vi "init_memtest_1channel_justNoise_v02.vi"(6 "memtest":T1={"Samples to Read"=2000, "Rate (Hz)"=20000.0, "Amplitude (mV/pA)"=10.0, "Offset (mV/pA)"=0.0, "Frequency (Hz)"=10.0, "duty cycle (%)"=50.0, "phase"=90.0} {"phase" format="%.2p"; "duty cycle (%)" format="%0.2f"}, 8 "AO error in":errorcluster, 9 "AO physical channels":tag="cDAQ1Mod3/ao14", 10 "AI error in":errorcluster, 11 "AI Physical Channels":tag="cDAQ1Mod1/ai0") -> (0 "AO error out":errorcluster, 1 "AO task out":refnum<k21>, 2 "AI error out":errorcluster, 3 "AI task out":refnum<k21>, 4 "view memtest":waveform(dbl)(graph))   [LabVIEW 2015]
uses:
  <vilib>/DAQmx/configure/timing.llb/DAQmx Timing (Sample Clock).vi
  <vilib>/DAQmx/create/channels.llb/DAQmx Create Channel (AI-Voltage-Basic).vi
  <vilib>/DAQmx/create/channels.llb/DAQmx Create Channel (AO-Voltage-Basic).vi
  <vilib>/DAQmx/configure/trigger.llb/DAQmx Start Trigger (Digital Edge).vi
  <vilib>/DAQmx/write.llb/DAQmx Write (Analog Wfm 1Chan NSamp).vi
  controls/memtest_def.ctl
panel:
  out "command memtest 2":waveform(dbl)(graph)
  out "command memtest":waveform(dbl)(graph)
  in  "which clamp":enum16{"VClamp", "IClamp"}(ring)
  # "init memtest"
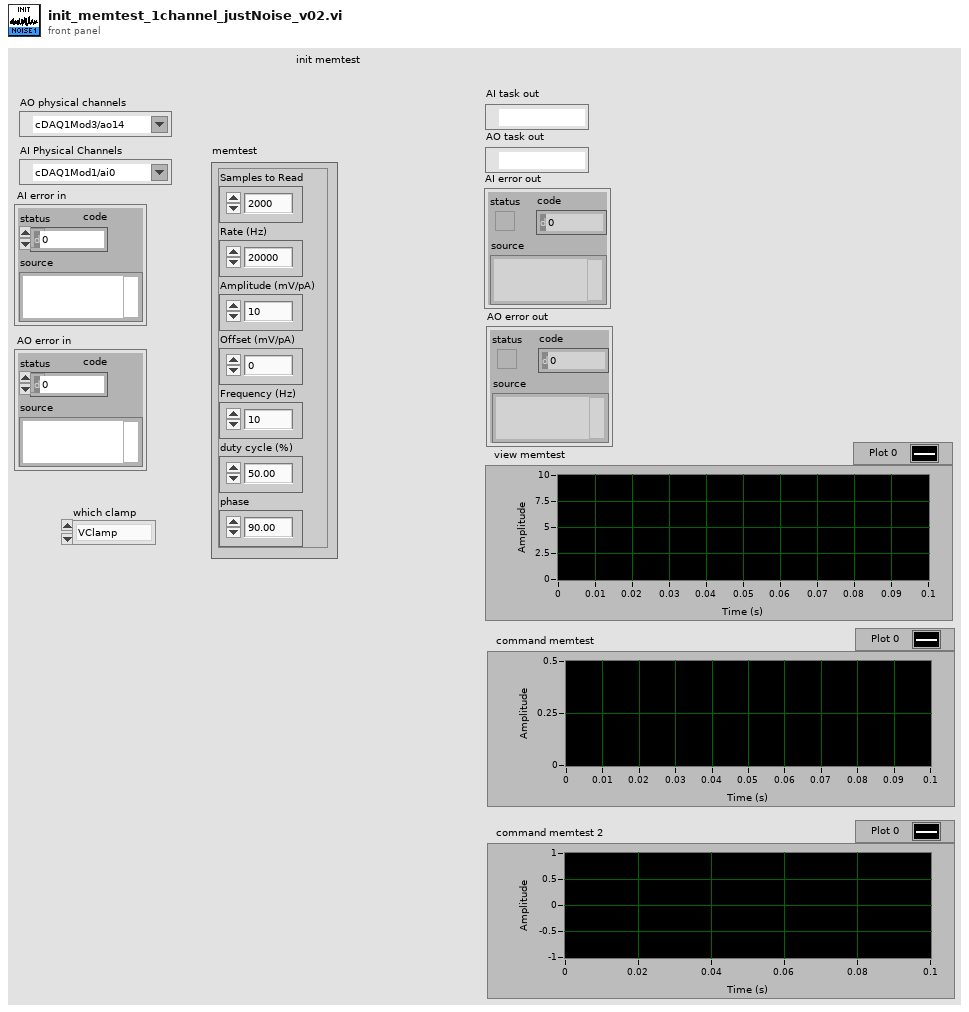
[diagram p1: front panel]
types:
  T1 = typedef "memtest_def.ctl" = cluster{"Samples to Read":i32, "Rate (Hz)":dbl, "Amplitude (mV/pA)":dbl, "Offset (mV/pA)":dbl, "Frequency (Hz)":dbl, "duty cycle (%)":dbl, "phase":dbl}
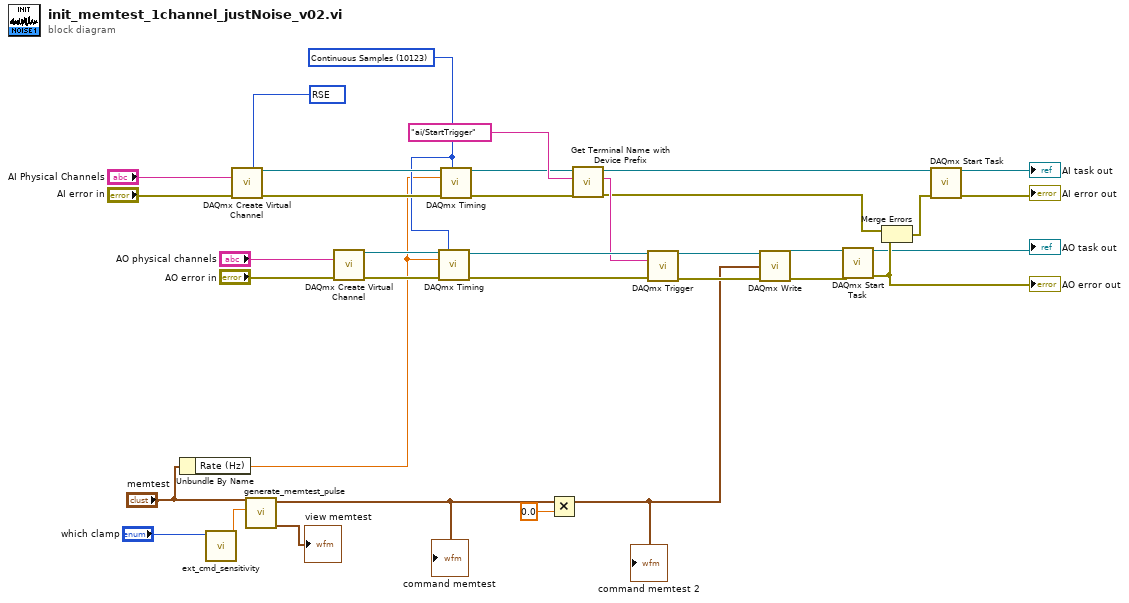
[diagram p0: block diagram]
diagram:
  w32 = 10083 items=["default"=-1, "RSE"=10083, "NRSE"=10078, "Differential"=10106, "Pseudodifferential"=12529] ("input terminal configuration")
  w23 = 10123 items=["Finite Samples"=10178, "Continuous Samples"=10123] ("sample mode")
  n1 = Unbundle By Name("memtest") -> ("Rate (Hz)"=w7:dbl)
  n2 = call "ext_cmd_sensitivity.vi"("which clamp"="which clamp") -> ("division factor"=w5:dbl)  [unwired: 10 in]
  n3 = call-poly <vilib>:"DAQmx Create Virtual Channel.vi"("input terminal configuration"=w32, "physical channels"="AI Physical Channels", "error in"="AI error in") -> ("task out"=w34:refnum<k21>, "error out"=w35:errorcluster)  [unwired: 11 in]
  n4 = call "generate_memtest_pulse.vi"("external cmd sensitivity"=w5, "memtest"="memtest") -> ("view memtest"=→"view memtest":waveform(dbl), "command memtest"=w4:waveform(dbl))  [unwired: 8 in]
  "command memtest" <- w4
  n5 = call-poly <vilib>:"DAQmx Create Virtual Channel.vi"("physical channels"="AO physical channels", "error in"="AO error in") -> ("task out"=w25:refnum<k21>, "error out"=w24:errorcluster)  [unwired: 12 in]
  n6 = call-poly <vilib>:"DAQmx Timing.vi"("task/channels in"=w25, "sample mode"=w23, "rate"=w7, "error in"=w24) -> ("task out"=w21:refnum<k21>, "error out"=w22:errorcluster)  [unwired: 10 in]
  n7 = call-poly <vilib>:"DAQmx Timing.vi"("task/channels in"=w34, "sample mode"=w23, "rate"=w7, "error in"=w35) -> ("task out"=w29:refnum<k21>, "error out"=w28:errorcluster)  [unwired: 10 in]
  n8 = Multiply(x=w4, y=0.0) -> (x*y=w2:waveform(dbl))
  "command memtest 2" <- w2
  n9 = call "Get Terminal Name with Device Prefix.vi"("error in (no error)"=w28, "Local Terminal Name"="ai/StartTrigger" ("terminal"), "task/channels in"=w29) -> ("error out"=w17:errorcluster, "Terminal Name with Device Prefix"=w20:tag, "task out"=w12:refnum<k21>)  [unwired: 6 in]
  n10 = call-poly <vilib>:"DAQmx Trigger.vi"("task/channels in"=w21, "source"=w20, "error in"=w22) -> ("task out"=w19:refnum<k21>, "error out"=w18:errorcluster)  [unwired: 11 in]
  n11 = call-poly <vilib>:"DAQmx Write.vi"("task/channels in"=w19, "data"=w2, "error in"=w18) -> ("task out"=w14:refnum<k21>, "error out"=w13:errorcluster)  [unwired: 10 in, 1 out]
  n12 = call <vilib>:"DAQmx Start Task.vi"("task/channels in"=w14, "error in"=w13) -> ("task out"=→"AO task out":refnum<k21>, "error out"=w15:errorcluster)  [unwired: 12 in]
  "AO error out" <- w15
  n13 = Merge Errors(w17, w15) -> (w16:errorcluster)
  n14 = call <vilib>:"DAQmx Start Task.vi"("task/channels in"=w12, "error in"=w16) -> ("task out"=→"AI task out":refnum<k21>, "error out"=→"AI error out":errorcluster)  [unwired: 12 in]
